vi "Get_Processed_Bytes_From_Data_Packet.vi"(8 "error in (no error)":errorcluster, 10 "Frame ID":u8, 11 "Node ID":u8) -> (0 "error out":errorcluster, 3 "Processed Bytes":u8[](array[numeric]))   [LabVIEW 2017]
uses:
  Controls/Data Packets/Data_Packet_FGV_Commands.ctl
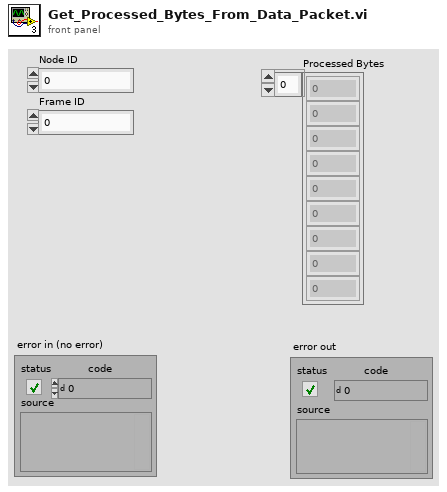
[diagram p1: front panel]
types:
  T1 = typedef "Data_Packet_FGV_Commands.ctl" = enum16{"Update Packet", "Load", "Read Packet Parameters", "Write Packet Parameters", "Read Packet Parameter", "Write Packet Parameter", "Read Data Packets", "Read Data Packet", "Read Data Packet by Parameter Name", "Get Parameter Node and Frame ID", "Read Data Packet from Node ID and Frame ID"}
  T2 = typedef "Data_Packet.ctl" = cluster{"Packet":T3, "Parameters":T7[]}
  T3 = typedef "Packet.ctl" = cluster{"Raw Bytes":u8[], "Checksum":bool, "Direction":T4, "Processed Bytes":u8[], "Node ID":u8, "Packet type":T5, "Frame Data":u32, "Priority":T6, "Frame ID":u8}
  T4 = typedef "Packet_Direction.ctl" = enum16{"Transmit", "Receive", "Bidirectional"}
  T5 = typedef "Packet_Type.ctl" = enum16{"Data", "Connection Management", "Remote Request", "Error/Status"}
  T6 = typedef "Packet_Priority.ctl" = enum16{"LOW", "HIGH"}
  T7 = typedef "Parameter.ctl" = cluster{"Parameter name":string, "Node name":string, "Node ID":u8, "Frame name":string, "Frame ID":u8, "Data type":T8, "Start Bit":i32, "Bit Length":i32, "Factor":dbl, "Offset":dbl, "Minimum":dbl, "Maximum":dbl, "Descriptor":string, "Enum values":string[], "Value":string}
  T8 = typedef "Parameter_Data_Type.ctl" = enum16{"BOOL", "UNSIGNED", "SIGNED", "FLOAT32", "ENUM"}
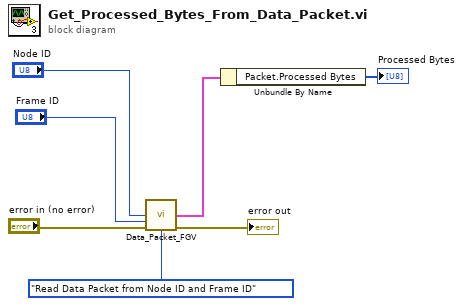
[diagram p0: block diagram]
diagram:
  n1 = call "Data_Packet_FGV.vi"("Node ID"="Node ID", "Frame ID"="Frame ID", "error in (no error)"="error in (no error)", "Commands"=Data_Packet_FGV_Commands."Read Data Packet from Node ID and Frame ID") -> ("Data_Packet Out"=w3:T2, "error out"=→"error out":errorcluster)  [unwired: 6 in, 4 out]
  n2 = Unbundle By Name(w3) -> ("Packet.Processed Bytes"=→"Processed Bytes":u8[])
